vi "H5Pget_fapl_multi.vi"(8 "error in (no error)":errorcluster, 11 "HDF5 Property List Ref":T1) -> (0 "error out":errorcluster, 1 "Member Name":string, 2 "Member FAPL":T1, 3 "HDF5 Property List Ref out":T1, 4 "Member Address":u64, 5 "Member":i32(ring) items=["H5FD_MEM_NOLIST"=-1, "H5FD_MEM_DEFAULT"=0, "H5FD_MEM_SUPER"=1, "H5FD_MEM_BTREE"=2, "H5FD_MEM_DRAW"=3, "H5FD_MEM_GHEAP"=4, "H5FD_MEM_LHEAP"=5, "H5FD_MEM_OHDR"=6], 6 "Relax":bool)   [LabVIEW 2017]
doc: "Returns information about the multi-file access property list."
uses:
  <vilib>/UPVI/lvhdf5/library.llb/HDF5 Ref.ctl
  <vilib>/UPVI/lvhdf5/h5helper.dll
panel:
  # "LVHDF5 Toolkit\nCopyright (c) 2005-2013 by Jason D. Sommerville\nCopyright (c) 2014 by UPVI, LLC.\n\nThis use and distribution of this file is governed by the terms found in \nLICENSE.txt distributed with this toolkit and installed at\n <user.lib>\\_lvhdf5\\LICENSE.txt"
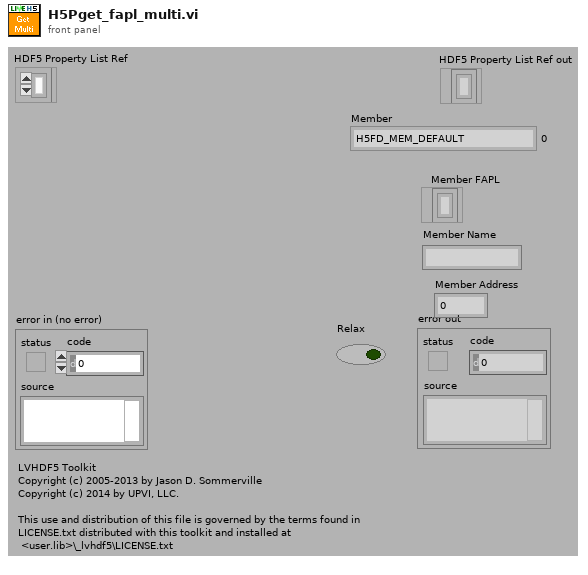
[diagram p1: front panel]
types:
  T1 = typedef "HDF5 Ref.ctl" = refnum<k1>
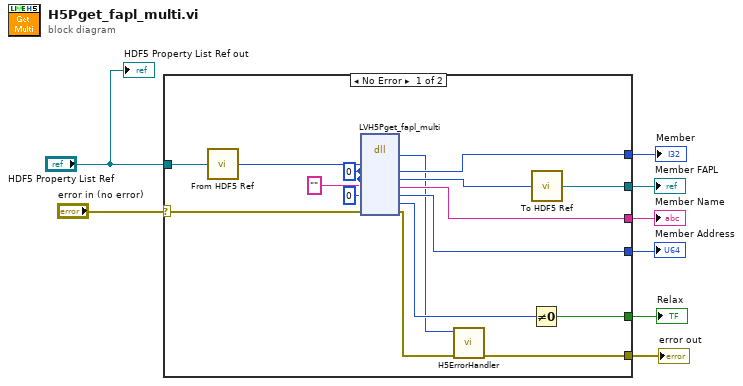
[diagram p0: block diagram]
diagram:
  n1 = case shown="No Error" "error in (no error)" {
    selector: "error in (no error)" -> [w14 w25]
    tunnel: [w10 w25] -> w7
    tunnel: "HDF5 Property List Ref" -> [w13 _]
    tunnel: [w22 _] -> w5
    tunnel: [w21 _] -> w4
    tunnel: [w18 _] -> w3
    tunnel: [w12 _] -> w2
    tunnel: [w16 _] -> w1
    frame No Error {
      w20 = 0 ("memb_map")
      n2 = call <vilib>:"From HDF5 Ref.vi"("HDF5 Ref"=w13) -> ("I32"=w24:i32)
      n3 = dll-call lib="C:/Program Files/National Instruments/LabVIEW 2017/vi.lib/UPVI/lvhdf5/h5helper.dll" fn="LVH5Pget_fapl_multi" label="H5Pget_fapl_multi"("plist_id"=w24, "memb_map"=w20, "memb_fapl"=w20, "memb_name"="", "memb_addr"=u64 0, "relax"=w20, "error"=w14) -> ("return type"=w9:i32, "memb_map"=w21:i32, "memb_fapl"=w23:i32, "memb_name"=w18:string, "memb_addr"=w12:u64, "relax"=w17:i32, "error"=w11:errorcluster)  [unwired: 4 in, 2 out]
      n4 = call <vilib>:"H5ErrorHandler.vi"("error in (no error)"=w11, "herr_t"=w9) -> ("error out"=w10:errorcluster)  [unwired: 3 in, 4 out]
      n5 = Not Equal To 0?(x=w17) -> (x != 0?=w16:bool)
      n6 = call <vilib>:"To HDF5 Ref.vi"("I32"=w23) -> ("HDF5 Ref"=w22:T1)
    }
    frame Error {
    }
  }
  "error out" <- w7
  "Member" <- w4
  "Member FAPL" <- w5
  "Member Name" <- w3
  "Member Address" <- w2
  "Relax" <- w1
  "HDF5 Property List Ref out" <- "HDF5 Property List Ref"
